vi "Edit Target Settings.vi"(8 "error in (no error)":errorcluster, 9 "Settings":T1={"Target Type"="", "IPAddress"="localhost", "PrimaryControlLoopProcessor (-2 is Automatic)"=-2, "DataProcessingLoopProcessor (-2 is Automatic)"=1, "DataProcessingLoopDecimation"=1, "DAQDigitalLinesDecimation"=512, "MaximumStreamedChannels"=0, "ExecutionMode"=0, "FilterDAQErrors"=FALSE, "FilterWatchdogErrors"=FALSE, "FPGAScanInterfaceMode"=0, "TargetRate"=0.0} {"FPGAScanInterfaceMode" items=["Use Current", "FPGA Mode", "Scan Mode"]; "ExecutionMode" items=["Parallel", "LowLatency"]}, 10 "System Definition Node Path":string, 11 "SysDef Ref":T3) -> (0 "error out":errorcluster, 2 "New Node Path":string, 3 "SysDef Ref Out":T3)   [LabVIEW 2019, in "Simple SysDef API.lvlib"]
uses:
  <userlib>/SimpleSysDef/Simple SysDef API.lvlib
  NationalInstruments.VeriStand.SystemDefinitionAPI
  <userlib>/SimpleSysDef/_SubVIs/System Definition Reference.ctl
  <userlib>/SimpleSysDef/_SubVIs/Edit Target Settings_Settings.ctl
  <userlib>/SimpleSysDef/_SubVIs/Add Target_Types.ctl
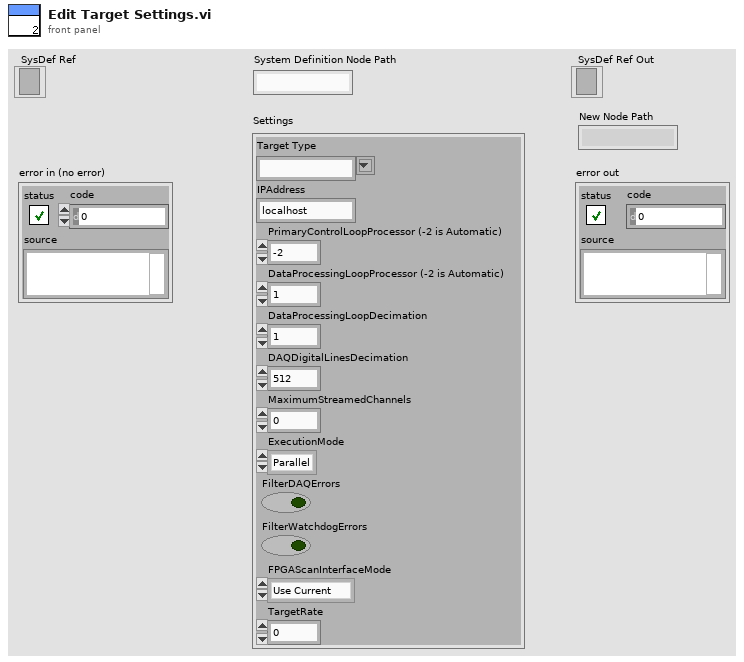
[diagram p1: front panel]
types:
  T1 = typedef "Simple SysDef API.lvlib/Edit Target Settings_Settings.ctl" = cluster{"Target Type":T2, "IPAddress":string, "PrimaryControlLoopProcessor (-2 is Automatic)":i32, "DataProcessingLoopProcessor (-2 is Automatic)":i32, "DataProcessingLoopDecimation":i32, "DAQDigitalLinesDecimation":u32, "MaximumStreamedChannels":i32, "ExecutionMode":i32, "FilterDAQErrors":bool, "FilterWatchdogErrors":bool, "FPGAScanInterfaceMode":u16, "TargetRate":dbl}
  T2 = typedef "Simple SysDef API.lvlib/Add Target_Types.ctl" = string
  T3 = typedef "Simple SysDef API.lvlib/System Definition Reference.ctl" = refnum<k24>
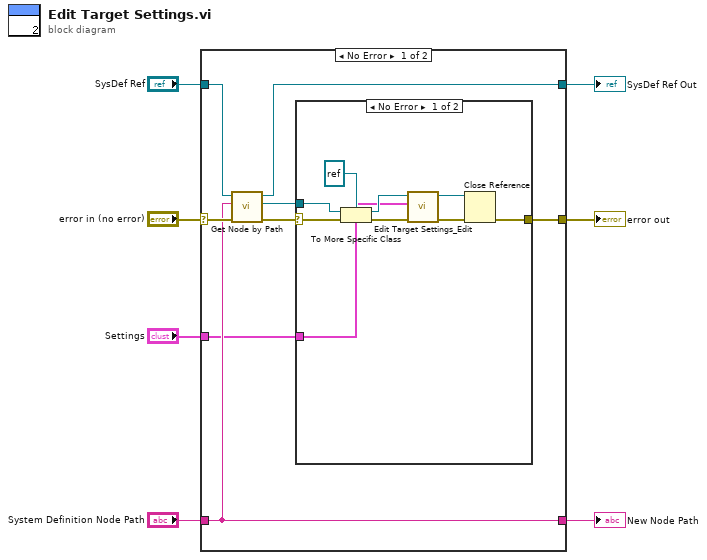
[diagram p0: block diagram]
diagram:
  n1 = case shown="No Error" "error in (no error)" {
    selector: "error in (no error)" -> [w15 w27]
    tunnel: [w12 w27] -> w6
    tunnel: "SysDef Ref" -> [w14 w26]
    tunnel: [w13 w26] -> w4
    tunnel: "System Definition Node Path" -> [w9 _]
    tunnel: "Settings" -> [w8 _]
    tunnel: [w9 _] -> w1
    frame No Error {
      n2 = call <userlib>:"Get Node by Path.vi"("error in (no error)"=w15, "System Definition Node Path"=w9, "SysDef Ref"=w14) -> ("error out"=w10:errorcluster, "Node Ref"=w11:refnum<k24>, "SysDef Ref Out"=w13:T3)  [unwired: 6 in]
      n3 = case shown="No Error" w10 {
        selector: w10 -> [w23 w25]
        tunnel: [w22 w25] -> w12
        tunnel: w11 -> [w24 _]
        tunnel: w8 -> [w16 _]
        frame No Error {
          n4 = To More Specific Class(target class=refnum<k24> refnum ("Node Ref"), reference=w24, error in=w23) -> (specific class reference=w18:refnum<k24>, error out=w20:errorcluster)
          n5 = call <userlib>:"Edit Target Settings_Edit.vi"("error in (no error)"=w20, "Settings"=w16, "Target Ref"=w18) -> ("error out"=w19:errorcluster, "Target Ref Out"=w17:refnum<k24>)  [unwired: 7 in]
          n6 = Close Reference(reference=w17, error in (no error)=w19) -> (error out=w22:errorcluster)
        }
        frame Error {
        }
      }
    }
    frame Error {
    }
  }
  "SysDef Ref Out" <- w4
  "error out" <- w6
  "New Node Path" <- w1
